vi "Battery AD Counts.vi"(6 "Message":string, 8 "Ready Button":bool) -> (0 "Batt280":i32, 3 "Batt320":i32)   [LabVIEW 2013]
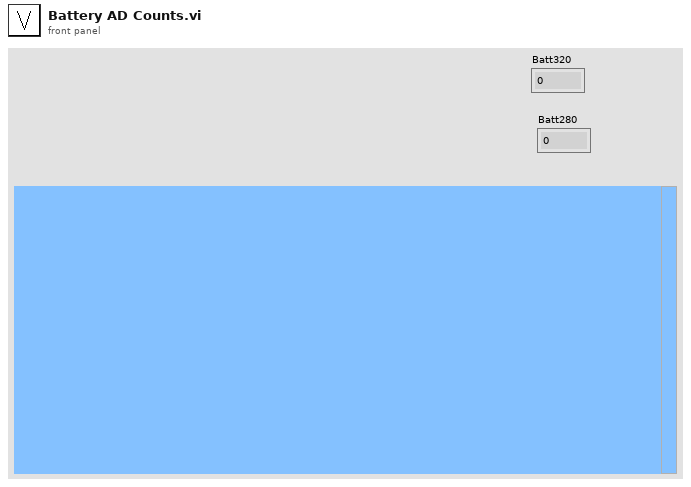
[diagram p1: front panel]
types:
  T1 = enum8{"Enabled", "Disabled", "Disabled and Grayed Out"}
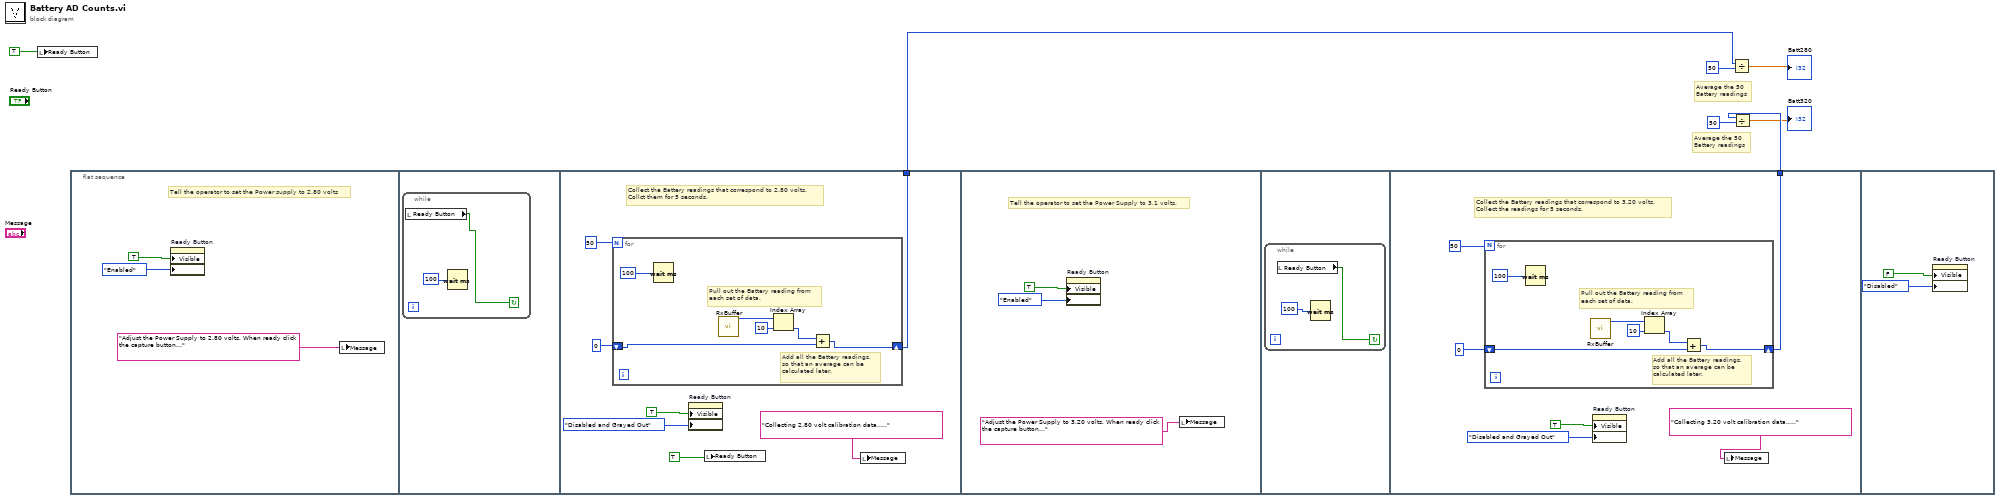
[diagram p0: block diagram]
diagram:
  # "Average the 50 \nBattery readings"
  # "Average the 50 \nBattery readings"
  n1 = local write "Ready Button"(TRUE) -> ()
  n2 = flat-sequence {
    tunnel: [w17] -> w6
    tunnel: [w35] -> w4
    frame #0 {
      # "Tell the operator to set the Power supply to 2.80 volts"
      n3 = property on="Ready Button" class="Bool (strict)"("Visible"=TRUE, "DisabledEnum"=T1."Enabled" ("Disabled")) -> ()  [unwired: 2 in, 2 out]
      n4 = local write "Message"("Adjust the Power Supply to 2.80 volts. When ready click the capture button..." ("Message")) -> ()
    }
    frame #1 {
      n5 = while {
        stop <- w11 continue-if-true
        n6 = local read "Ready Button"() -> (w11:bool)
        n7 = Wait (ms)(milliseconds to wait=u32 100) -> ()  [unwired: 1 out]
      }
    }
    frame #2 {
      # "Collect the Battery readings that correspond to 2.80 volts.\nCollct them for 5 seconds."
      n8 = for {
        N: 50 -> [_]
        shift-right: [w20] -> w17
        shift-left: u64 0 -> [w22]
        # "Add all the Battery readings, \nso that an average can be \ncalculated later."
        # "Pull out the Battery reading from\neach set of data."
        n9 = Wait (ms)(milliseconds to wait=u32 100) -> ()  [unwired: 1 out]
        n10 = call "RxBuffer.vi"() -> ("RxData Out"=w24:u16[])  [unwired: 10 in, 9 out]
        n11 = Index Array(array=w24, index=10) -> (element=w21:u16)
        n12 = Add(x=w21, y=w22) -> (x+y=w20:u64)
      }
      n13 = property on="Ready Button" class="Bool (strict)"("Visible"=TRUE, "DisabledEnum"=T1."Disabled and Grayed Out" ("Disabled")) -> ()  [unwired: 2 in, 2 out]
      n14 = local write "Ready Button"(TRUE) -> ()
      n15 = local write "Message"("Collecting 2.80 volt calibration data....." ("Message")) -> ()
    }
    frame #3 {
      # "Tell the operator to set the Power Supply to 3.1 volts."
      n16 = property on="Ready Button" class="Bool (strict)"("Visible"=TRUE, "DisabledEnum"=T1."Enabled" ("Disabled")) -> ()  [unwired: 2 in, 2 out]
      n17 = local write "Message"("Adjust the Power Supply to 3.20 volts. When ready click the capture button..." ("Message")) -> ()
    }
    frame #4 {
      n18 = while {
        stop <- w29 continue-if-true
        n19 = local read "Ready Button"() -> (w29:bool)
        n20 = Wait (ms)(milliseconds to wait=u32 100) -> ()  [unwired: 1 out]
      }
    }
    frame #5 {
      # "Collect the Battery readings that correspond to 3.20 volts.\nCollect the readings for 5 seconds."
      n21 = for {
        N: 50 -> [_]
        shift-right: [w37] -> w35
        shift-left: u64 0 -> [w39]
        # "Add all the Battery readings, \nso that an average can be \ncalculated later."
        # "Pull out the Battery reading from\neach set of data."
        n22 = Wait (ms)(milliseconds to wait=u32 100) -> ()  [unwired: 1 out]
        n23 = call "RxBuffer.vi"() -> ("RxData Out"=w41:u16[])  [unwired: 10 in, 9 out]
        n24 = Index Array(array=w41, index=10) -> (element=w38:u16)
        n25 = Add(x=w38, y=w39) -> (x+y=w37:u64)
      }
      n26 = property on="Ready Button" class="Bool (strict)"("Visible"=TRUE, "DisabledEnum"=T1."Disabled and Grayed Out" ("Disabled")) -> ()  [unwired: 2 in, 2 out]
      n27 = local write "Message"("Collecting 3.20 volt calibration data....." ("Message")) -> ()
    }
    frame #6 {
      n28 = property on="Ready Button" class="Bool (strict)"("Visible"=FALSE, "DisabledEnum"=T1."Disabled" ("Disabled")) -> ()  [unwired: 2 in, 2 out]
    }
  }
  n29 = Divide(x=w6, y=u64 50) -> (x/y=→"Batt280":dbl)
  n30 = Divide(x=w4, y=u64 50) -> (x/y=→"Batt320":dbl)
